vi "GetTachometersProperties.vi"(8 "error in (no error)":errorcluster, 9 "settling time (seconds)":dbl, 10 "channel properties":T1[](array[typedef]), 11 "channel type":string) -> (0 "error out":errorcluster, 3 "tachometer":T2)   [LabVIEW 2017, in "CmsVirtualChannel.lvlib"]
uses:
  <vilib>/addons/InsightCM/Devices/Shared/Cms/CmsVirtualChannel/CmsVirtualChannel.lvlib
  <vilib>/addons/InsightCM/Devices/Shared/Cms/CmsVirtualChannel/controls/Tachometer.ctl
  <vilib>/addons/InsightCM/Utilities/Analysis/Vibration/controls/Tachometer.ctl
  <vilib>/addons/InsightCM/Utilities/Analysis/Vibration/controls/DigitalTachometer.ctl
  <vilib>/addons/InsightCM/MessageBus/Base/controls/KeyValuePair.ctl
  <vilib>/addons/InsightCM/Utilities/PropertyHelpers/PropertyHelpers.lvlib
  <vilib>/addons/InsightCM/Utilities/Analysis/Vibration/VibrationAnalysisFunctions.lvlib
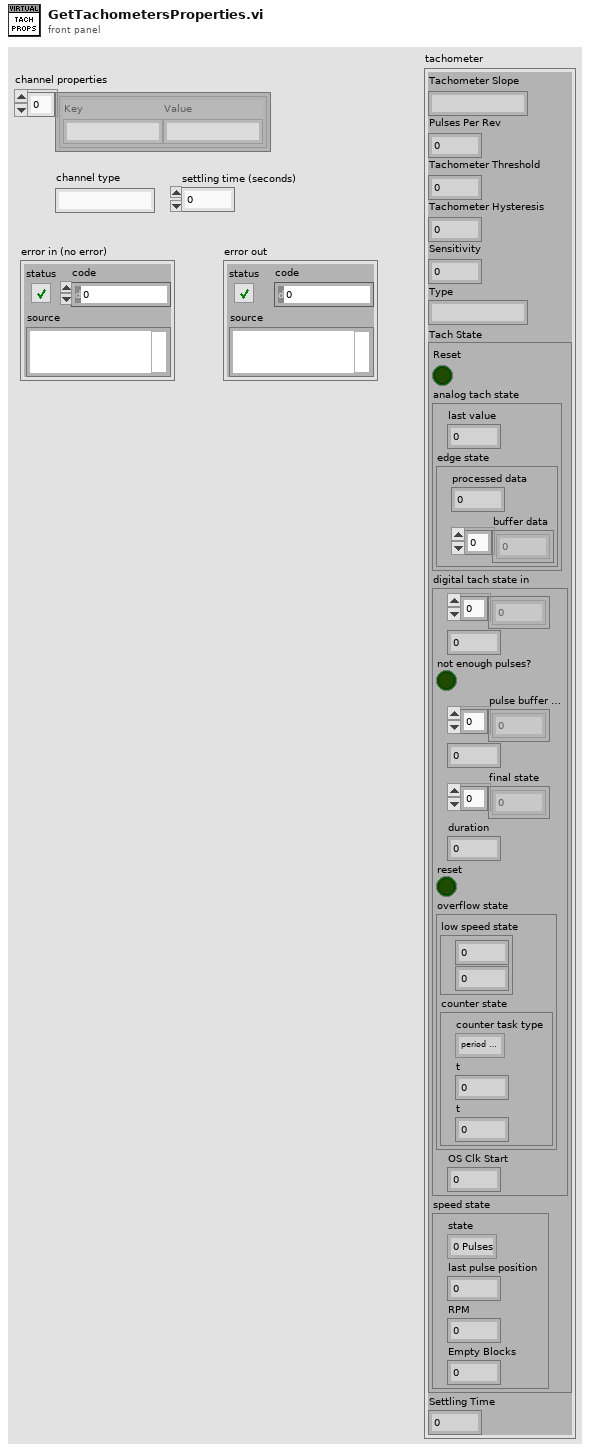
[diagram p1: front panel]
types:
  T1 = typedef "KeyValuePair.ctl" = cluster{"Key":string, "Value":string}
  T2 = typedef "CmsVirtualChannel.lvlib/Tachometer.ctl" = cluster{"Tachometer Slope":string, "Pulses Per Rev":i32, "Tachometer Threshold":dbl, "Tachometer Hysteresis":dbl, "Sensitivity":dbl, "Type":string, "Tach State":T3, "Settling Time":dbl}
  T3 = typedef "VibrationAnalysisFunctions.lvlib/Tachometer.ctl" = cluster{"Reset":bool, "analog tach state":cluster{"last value":dbl, "edge state":cluster{"processed data":dbl, "buffer data":dbl[]}}, "digital tach state in":T4, "speed state":cluster{"state":enum16{"0 Pulses", "1 Pulse", "2+ Pulses"}, "last pulse position":dbl, "RPM":dbl, "Empty Blocks":i32}}
  T4 = typedef "VibrationAnalysisFunctions.lvlib/DigitalTachometer.ctl" = cluster{dbl[], i32, "not enough pulses?":bool, "pulse buffer out":dbl[], i32, "final state":dbl[], "duration":dbl, "reset":bool, "overflow state":cluster{"low speed state":cluster{dbl, ext}, "counter state":cluster{"counter task type":enum16{"period measurement", "event counting"}, "t":dbl, "t":dbl}}, "OS Clk Start":dbl}
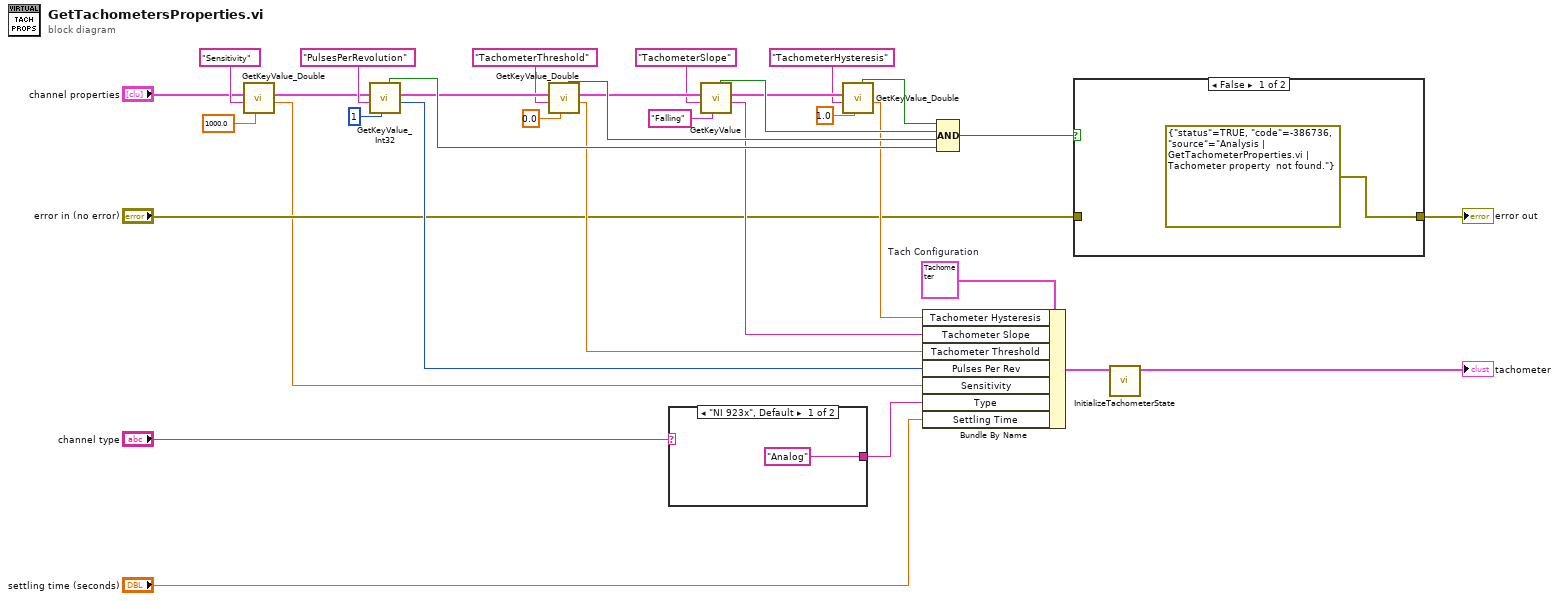
[diagram p0: block diagram]
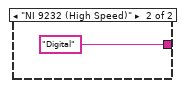
[diagram p2: hidden frame]
diagram:
  w33 = T2 {"Tachometer Slope"="", "Pulses Per Rev"=0, "Tachometer Threshold"=0.0, "Tachometer Hysteresis"=0.0, "Sensitivity"=0.0, "Type"="", "Tach State"={"Reset"=FALSE, "analog tach state"={"last value"=0.0, "edge state"={"processed data"=0.0, "buffer data"=[]}}, "digital tach state in"={[], 0, "not enough pulses?"=FALSE, "pulse buffer out"=[], 0, "final state"=[], "duration"=0.0, "reset"=FALSE, "overflow state"={"low speed state"={0.0, 0.0}, "counter state"={"counter task type"=enum."period measurement", "t"=0.0, "t"=0.0}}, "OS Clk Start"=0.0}, "speed state"={"state"=enum."0 Pulses", "last pulse position"=0.0, "RPM"=0.0, "Empty Blocks"=0}}, "Settling Time"=0.0}  # Tach Configuration
  n1 = call <vilib>:"GetKeyValue_Double.vi"("default"=1000.0, "key"="Sensitivity" ("name"), "key value pairs"="channel properties") -> ("value"=w4:dbl, "key value pairs out"=w6:T1[])  [unwired: 6 in, 1 out]
  n2 = call <vilib>:"GetKeyValue_Int32.vi"("default"=1, "key"="PulsesPerRevolution" ("name"), "key value pairs"=w6) -> ("value"=w16:i32, "key value pairs out"=w24:T1[], "found"=w26:bool)  [unwired: 6 in]
  n3 = call <vilib>:"GetKeyValue_Double.vi"("default"=0.0, "key"="TachometerThreshold" ("name"), "key value pairs"=w24) -> ("value"=w15:dbl, "key value pairs out"=w23:T1[], "found"=w27:bool)  [unwired: 6 in]
  n4 = case shown="\"NI 923x\", Default" "channel type" {
    tunnel: ["Analog" "Digital"] -> w2
    frame "NI 923x", Default {
    }
    frame "NI 9232 (High Speed)" {
    }
  }
  n5 = call <vilib>:"GetKeyValue.vi"("default value"="Falling", "key"="TachometerSlope" ("name"), "key value pairs"=w23) -> ("value"=w18:string, "key value pairs out"=w22:T1[], "found"=w28:bool)  [unwired: 6 in]
  n6 = call <vilib>:"GetKeyValue_Double.vi"("default"=1.0, "key"="TachometerHysteresis" ("name"), "key value pairs"=w22) -> ("value"=w14:dbl, "found"=w29:bool)  [unwired: 6 in, 1 out]
  n7 = Bundle By Name(cluster=w33, "Tachometer Hysteresis"=w14, "Tachometer Slope"=w18, "Tachometer Threshold"=w15, "Pulses Per Rev"=w16, "Sensitivity"=w4, "Type"=w2, "Settling Time"="settling time (seconds)") -> (w32:T2)
  n8 = Compound Arithmetic op=AND(w29, w28, w27, w26) -> (w25:bool)
  n9 = case shown="False" w25 {
    tunnel: [errorcluster {"status"=TRUE, "code"=-386736, "source"="Analysis | GetTachometerProperties.vi | Tachometer property  not found."} ("error in (no error)") w37] -> w30
    tunnel: "error in (no error)" -> [_ w37]
    frame False {
    }
    frame True {
    }
  }
  "error out" <- w30
  n10 = call <vilib>:"InitializeTachometerState.vi"("Tachometer in"=w32) -> ("Tachometer out"=→"tachometer":T2)  [unwired: 9 in, 1 out]
